vi "OP600ZP_PDU.vi"(8 "errin":errorcluster caption="entrée d'erreur (pas d'erreur)") -> (0 "errout":errorcluster caption="sortie d'erreur", 3 "PASS?":bool, 4 "ISO_PDU-":string, 6 "ISO_PDU+":string)   [LabVIEW 2020]
uses:
  OP500ZP_VGConf.vi
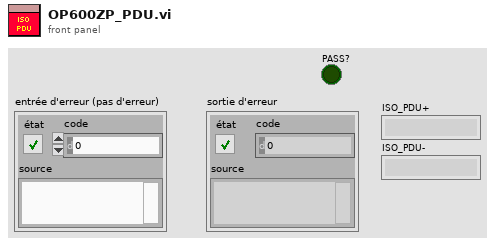
[diagram p1: front panel]
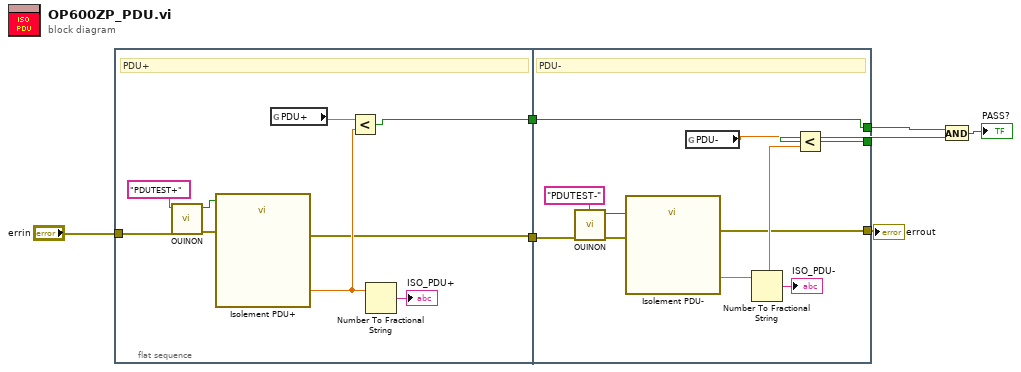
[diagram p0: block diagram]
diagram:
  n1 = flat-sequence {
    tunnel: "errin" -> [w16]
    tunnel: [w9] -> w3
    tunnel: [w8] -> w2
    tunnel: [w23] -> w6
    tunnel: [w19] -> w4
    tunnel: w3 -> [w18]
    tunnel: w2 -> [w17]
    tunnel: [w17] -> w1
    frame #0 {
      # "PDU+"
      n2 = call "OUINON.vi"("errin"=w16, "image"="PDUTEST+") -> ("error out"=w15:errorcluster, "OUI/NON"=w13:bool)  [unwired: 8 in]
      n3 = call "Isolement PDU+"("Enable"=w13, "error in (no error)"=w15) -> ("ISO_PDU+"=w12:dbl, "error out"=w9:errorcluster)  [unwired: 15 in, 1 out]
      n4 = global read "OP500ZP_VGConf.vi" "PDU+"() -> (w10:dbl)
      n5 = Less?(x=w10, y=w12) -> (x < y?=w8:bool)
      n6 = Number To Fractional String(number=w12) -> (F-format string=→"ISO_PDU+":string)  [unwired: 3 in]
    }
    frame #1 {
      # "PDU-"
      n7 = call "OUINON.vi"("errin"=w18, "image"="PDUTEST-") -> ("error out"=w25:errorcluster, "OUI/NON"=w24:bool)  [unwired: 8 in]
      n8 = call "Isolement PDU-"("Enable"=w24, "error in (no error)"=w25) -> ("ISO_PDU-"=w22:dbl, "error out"=w19:errorcluster)  [unwired: 15 in, 1 out]
      n9 = global read "OP500ZP_VGConf.vi" "PDU-"() -> (w20:dbl)
      n10 = Number To Fractional String(number=w22) -> (F-format string=→"ISO_PDU-":string)  [unwired: 3 in]
      n11 = Less?(x=w20, y=w22) -> (x < y?=w23:bool)
    }
  }
  n12 = And(x=w1, y=w6) -> (x .and. y?=→"PASS?":bool)
  "errout" <- w4
